vi "Wfm_rozmiar_do_skali.vi"(11 "Bufor in":T1) -> (3 "Size (s)":dbl)   [LabVIEW 2013]
doc: "pobiera długość wektora i parametr dT\npierwszego kanału analogowego i liczy rozmiar osi X wykresu"
uses:
  Kontrolki/Przetwarzanie/Kanaly.ctl
panel:
  out "error out":errorcluster
  in  "error in (no error)":errorcluster
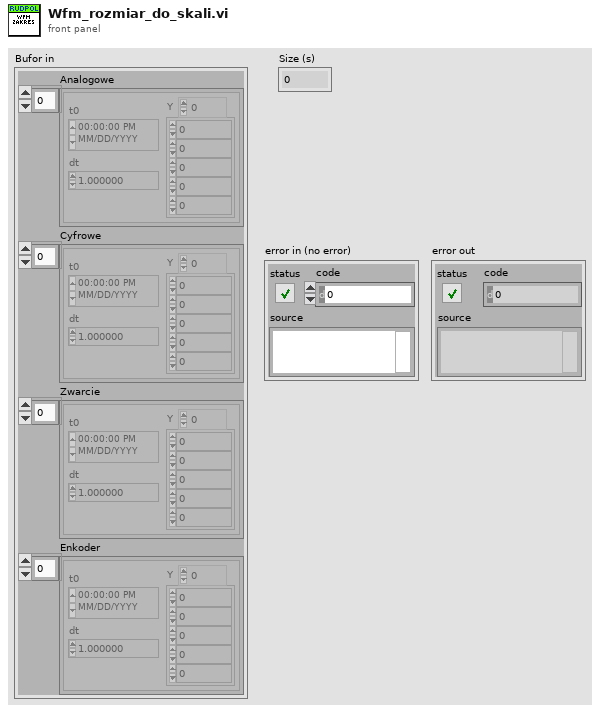
[diagram p1: front panel]
types:
  T1 = typedef "Kanaly.ctl" = cluster{"Analogowe":waveform(dbl)[], "Cyfrowe":waveform(dbl)[], "Zwarcie":waveform(dbl)[], "Enkoder":waveform(dbl)[]}
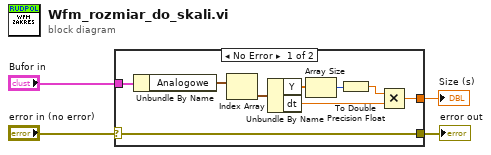
[diagram p0: block diagram]
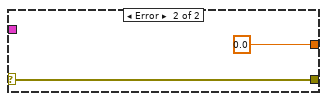
[diagram p2: hidden frame]
diagram:
  n1 = case shown="No Error" "error in (no error)" {
    selector: "error in (no error)" -> [w5 w14]
    tunnel: [w13 0.0] -> w4
    tunnel: "Bufor in" -> [w8 _]
    tunnel: [w5 w14] -> w1
    frame No Error {
      n2 = Unbundle By Name(w8) -> ("Analogowe"=w9:waveform(dbl)[])
      n3 = Index Array(array=w9) -> (element=w10:waveform(dbl))  [unwired: 1 in]
      n4 = Unbundle By Name(w10) -> ("Y"=w11:dbl[], "dt"=w12:dbl)
      n5 = Array Size(array=w11) -> (size(s)=w7:i32)
      n6 = To Double Precision Float(number=w7) -> (double precision float=w6:dbl)
      n7 = Multiply(x=w6, y=w12) -> (x*y=w13:dbl)
    }
    frame Error {
    }
  }
  "Size (s)" <- w4
  "error out" <- w1
